vi "Test_NotifyStop_ProcessFinalCopy_QueuedMessageExecuted.vi"(8 "error in (no error)":errorcluster, 11 "TestCase in":refnum<class "TestMessageCycle.lvclass">) -> (0 "error out":errorcluster, 3 "TestCase out":refnum<class "TestMessageCycle.lvclass">)   [LabVIEW 2017, in "TestMessageCycle.lvclass"]
uses:
  TestMessageCycle.lvclass
  Source/MessageCycle/Message Cycle Notifications.ctl
  Source/MessageCycle/MessageCycle.lvclass/MessageCycle.ctl
  <vilib>/ActorFramework/Message Enqueuer/Message Enqueuer.lvclass/Message Enqueuer.ctl
  df307ab6-d25a-4da9-84af-fd7a900fa043.vi
  a68a8fc0-880c-4d62-94bb-433110ca28ec.vi
  <vilib>/ActorFramework/Message Enqueuer/Enqueue.vi
  Doubles/MessageCountsExecutions/MessageCountsExecutions.lvclass
  C:/Program Files (x86)/National Instruments/LabVIEW 2017/vi.lib/ActorFramework/Message/Message.lvclass
  Doubles/ActorCountsMessageCycles/ActorCountsMessageCycles.lvclass
  C:/Program Files (x86)/National Instruments/LabVIEW 2017/vi.lib/ActorFramework/Actor/Actor.lvclass
  Source/MessageCycle/MessageCycle.lvclass
  <vilib>/ActorFramework/Stop Msg/Stop Msg.lvclass
  Source/MessageCycle/Launch Deferred Timeout Notifier.vi
  <vilib>/ActorFramework/Message Priority Queue/Priority Enqueue.vi
  <vilib>/ActorFramework/Message/Message.lvclass
  <vilib>/ActorFramework/Actor/Actor.lvclass
panel:
  out "Messages Executed":u32
  out "Cyclic Messages Received":u32
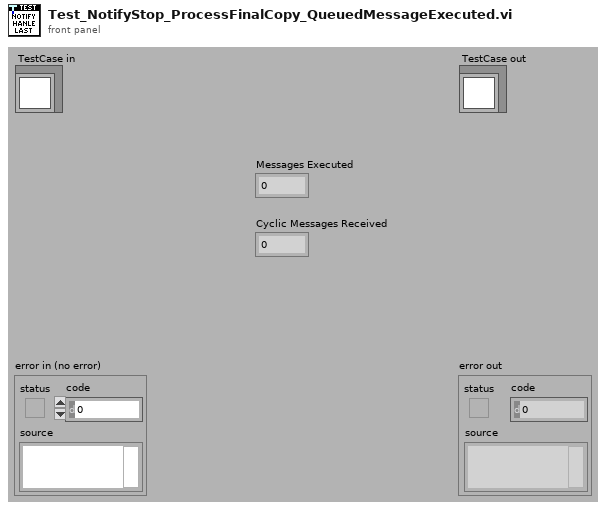
[diagram p1: front panel]
types:
  T1 = typedef "MessageCycle.lvclass/Message Cycle Notifications.ctl" = enum16{"Process Final Copy and Stop", "Stop Immediately", "Substitute Last Message and Stop"}
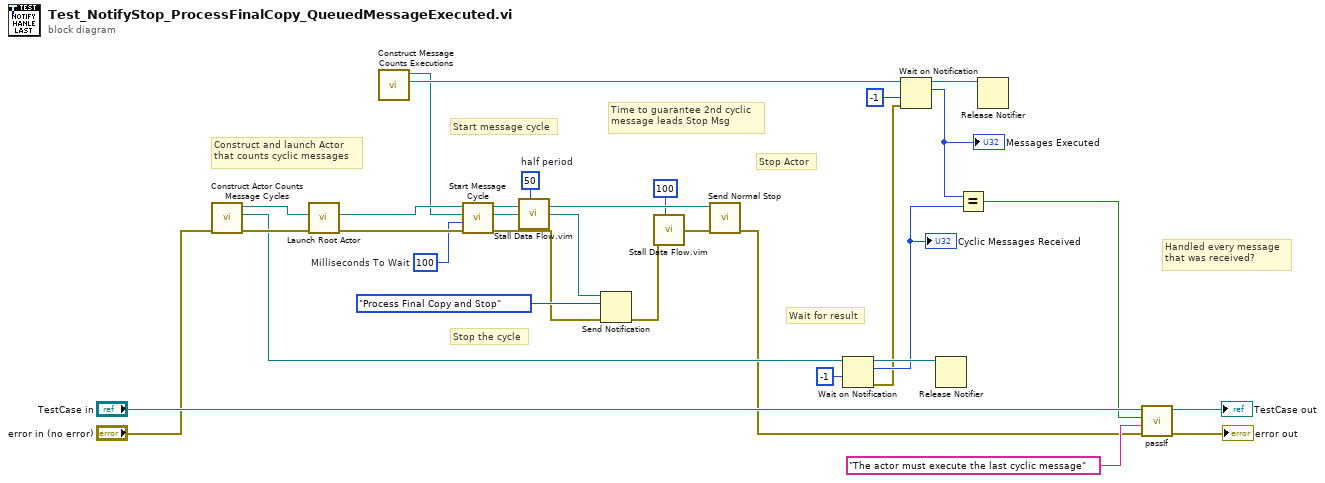
[diagram p0: block diagram]
diagram:
  w8 = u32 50  # half period
  w27 = 100  # Milliseconds To Wait
  # "Time to guarantee 2nd cyclic\nmessage leads Stop Msg"
  # "Stop the cycle"
  # "Wait for result"
  # "Stop Actor"
  # "Start message cycle"
  # "Handled every message\nthat was received?"
  # "Construct and launch Actor\nthat counts cyclic messages"
  n1 = call "Construct Actor Counts Message Cycles.vi"("error in (no error)"="error in (no error)") -> ("error out"=w20:errorcluster, "Final Count"=w19:refnum<notifier>, "ActorCountsMessageCycles"=w22:refnum<class "ActorCountsMessageCycles.lvclass">)  [unwired: 8 in]
  n2 = call <vilib>:"Launch Root Actor.vi"("error in (no error)"=w20, "Actor"=w22) -> ("error out"=w31:errorcluster, "Actor's Enqueuer"=w26:refnum<class "Message Enqueuer.lvclass">)  [unwired: 8 in]
  n3 = call "Construct Message Counts Executions.vi"() -> ("Message Executions"=w4:refnum<notifier>, "CyclicMessageCountsCycles out"=w1:refnum<class "MessageCountsExecutions.lvclass">)  [unwired: 9 in, 1 out]
  n4 = call "Start Message Cycle.vi"("error in (no error)"=w31, "Inter-Message Wait [ms] (0)"=w27, "Message"=w1, "Message Enqueuer"=w26) -> ("error out"=w11:errorcluster, "Message Cycle Notifier"=w14:refnum<notifier>, "Message Enqueuer out"=w25:refnum<class "Message Enqueuer.lvclass">)  [unwired: 5 in]
  n5 = call "Stall Data Flow.vim"("value in"=w14, "milliseconds to wait"=w8) -> ("value out"=w12:refnum<notifier>)  [unwired: 1 out]
  n6 = Send Notification(notification=Message_Cycle_Notifications."Process Final Copy and Stop", notifier=w12, error in (no error)=w11) -> (error out=w10:errorcluster)  [unwired: 1 out]
  n7 = call "Stall Data Flow.vim"("value in"=w10, "milliseconds to wait"=u32 100) -> ("value out"=w9:errorcluster)  [unwired: 1 out]
  n8 = call <vilib>:"Send Normal Stop.vi"("error in (no error)"=w9, "Message Enqueuer"=w25) -> ("error out"=w16:errorcluster)  [unwired: 9 in]
  n9 = Wait on Notification(notifier=w19, timeout in ms (-1)=-1) -> (notifier out=w17:refnum<notifier>, notification=w15:u32, error out=w2:errorcluster)  [unwired: 2 in, 1 out]
  "Cyclic Messages Received" <- w15
  n10 = Wait on Notification(notifier=w4, timeout in ms (-1)=-1, error in (no error)=w2) -> (notifier out=w6:refnum<notifier>, notification=w3:u32)  [unwired: 1 in, 2 out]
  "Messages Executed" <- w3
  n11 = Release Notifier(notifier=w17) -> ()  [unwired: 2 in, 3 out]
  n12 = Equal?(x=w3, y=w15) -> (x = y?=w24:bool)
  n13 = Release Notifier(notifier=w6) -> ()  [unwired: 2 in, 3 out]
  n14 = call-dynamic "passIf.vi"("error in (no error)"=w16, "message (\"\")"="The actor must execute the last cyclic message" ("message (\"\")"), "pass"=w24, "TestCase in"="TestCase in") -> ("error out"=→"error out":errorcluster, "TestCase out"=→"TestCase out":refnum<class "TestMessageCycle.lvclass">)  [unwired: 6 in]
